vi "reenvioSMS (SubVI).vi"(10 "Datos":T1={"Imei"="359772033694416", "Evento"="359772033694416", "Lat"="359772033694416", "Lon"="359772033694416", "F_H_eve"=timestamp(0 s since 1904-01-01), "F_H_rec"=timestamp(0 s since 1904-01-01)}) -> ()   [LabVIEW 2012]
uses:
  <vilib>/addons/database/Auxilliary.llb/DB Tools Cursor Type.ctl
  <vilib>/addons/database/Connection.llb/DB Tools Open Connec (Path).vi
  <vilib>/addons/database/Connection.llb/Conn Execute.vi
  <vilib>/addons/database/Recordset.llb/Rec Get Recordset Properties (R).vi
  <vilib>/addons/database/Recordset.llb/Rec Fetch String Data (R).vi
  <vilib>/addons/database/Recordset.llb/Rec Destroy - Connection.vi
  <vilib>/addons/database/NI_Database_API.lvlib
panel:
  out "SMS":string
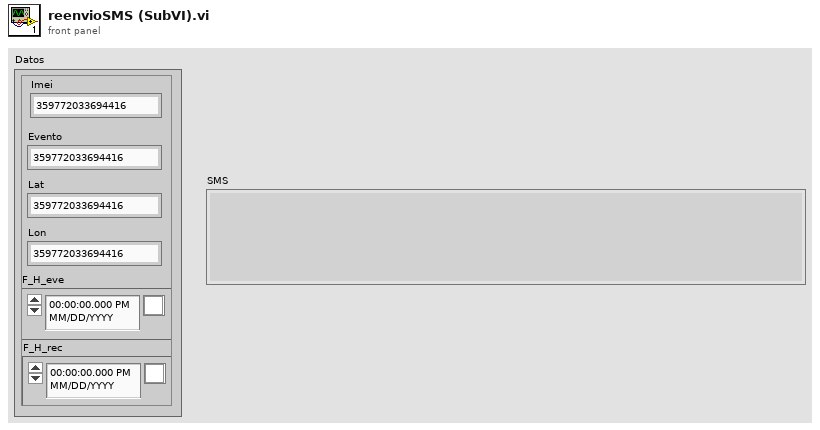
[diagram p1: front panel]
types:
  T1 = cluster{"Imei":string, "Evento":string, "Lat":string, "Lon":string, "F_H_eve":timestamp, "F_H_rec":timestamp}
  T2 = typedef "NI_Database_API.lvlib/DB Tools Cursor Type.ctl" = enum16{"forward-only", "keyset", "dynamic", "static"}
  T3 = enum16{"POC", "Imei", "Evento", "Lat", "Lon", "F_H_eve", "F_H_rec", "AVL_N", "AVL_pass", "Propietario", "Razon_Social", "Direccion", "Propietario_N", "Ciudad", "Marca", "Ruta", "N_Ruta", "Auditor", "Auditor_N"}
  T4 = typedef "NI_Database_API.lvlib/Conn ObjectReference.ctl" = refnum<k1>
  T5 = typedef "NI_Database_API.lvlib/Rec ObjectReference.ctl" = refnum<k1>
  T6 = enum16{"POC", "Imei", "Evento", "Lat", "Lon", "F_H_eve", "F_H_rec", "AVL_N", "AVL_pass", "Propietario", "Razon_Social", "Direccion", "Propietario_N", "Ciudad", "Marca", "Ruta", "N_Ruta", "Auditor_ST", "Auditor_P"}
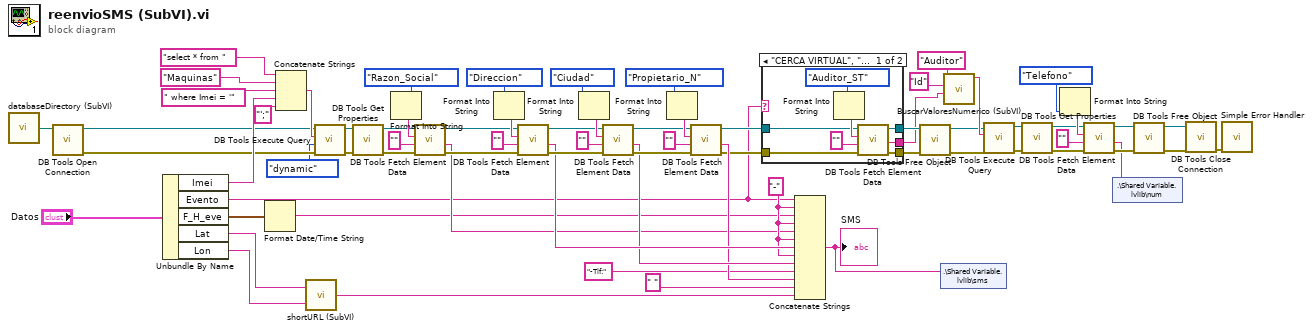
[diagram p0: block diagram]
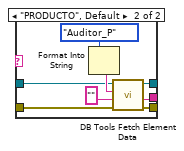
[diagram p2: hidden frame]
diagram:
  w41 = "-" ("type")
  n1 = call "databaseDirectory (SubVI).vi"() -> ("Application Directory"=w38:path)  [unwired: 1 in]
  n2 = call-poly <vilib>:"DB Tools Open Connection.vi"("connection information"=w38) -> ("error out"=w34:errorcluster, "connection reference"=w35:T4)  [unwired: 7 in]
  n3 = Unbundle By Name("Datos") -> ("Imei"=w36:string, "Evento"=w19:string, "F_H_eve"=w29:timestamp, "Lat"=w23:string, "Lon"=w22:string)
  n4 = Format Date/Time String(seconds (now)=w29) -> (date/time string=w28:string)  [unwired: 2 in]
  n5 = Concatenate Strings("select * from " ("SQL query"), "Maquinas" ("table"), " where Imei = '" ("Substring"), w36, "';") -> (w67:string)
  n6 = call "shortURL (SubVI).vi"("LON"=w22, "LAT"=w23) -> ("before substring"=w20:string)
  n7 = call-poly <vilib>:"DB Tools Execute Query.vi"("error in (no error)"=w34, "cursor type"=DB_Tools_Cursor_Type."dynamic", "SQL query"=w67, "connection reference"=w35) -> ("error out"=w68:errorcluster, "recordset reference"=w69:T5)  [unwired: 4 in]
  n8 = call-poly <vilib>:"DB Tools Get Properties.vi"("error in (no error)"=w68, "recordset reference"=w69) -> ("error out"=w26:errorcluster, "recordset reference out"=w27:T5)  [unwired: 3 in, 1 out]
  n9 = Format Into String(T3."Razon_Social") -> (resulting string=w61:string)  [unwired: 3 in, 1 out]
  n10 = call-poly <vilib>:"DB Tools Fetch Element Data.vi"("error in (no error)"=w26, "type"="", "column index"=w61, "recordset reference"=w27) -> ("error out"=w42:errorcluster, "data"=w40:string, "recordset reference out"=w56:T5)  [unwired: 3 in]
  n11 = Format Into String(T3."Direccion") -> (resulting string=w57:string)  [unwired: 3 in, 1 out]
  n12 = call-poly <vilib>:"DB Tools Fetch Element Data.vi"("error in (no error)"=w42, "type"="", "column index"=w57, "recordset reference"=w56) -> ("error out"=w52:errorcluster, "data"=w45:string, "recordset reference out"=w53:T5)  [unwired: 3 in]
  n13 = Format Into String(T3."Ciudad") -> (resulting string=w55:string)  [unwired: 3 in, 1 out]
  n14 = call-poly <vilib>:"DB Tools Fetch Element Data.vi"("error in (no error)"=w52, "type"="", "column index"=w55, "recordset reference"=w53) -> ("error out"=w50:errorcluster, "data"=w44:string, "recordset reference out"=w51:T5)  [unwired: 3 in]
  n15 = Format Into String(T3."Propietario_N") -> (resulting string=w60:string)  [unwired: 3 in, 1 out]
  n16 = call-poly <vilib>:"DB Tools Fetch Element Data.vi"("error in (no error)"=w50, "type"="", "column index"=w60, "recordset reference"=w51) -> ("error out"=w32:errorcluster, "data"=w43:string, "recordset reference out"=w33:T5)  [unwired: 3 in]
  n17 = case shown="\"CERCA VIRTUAL\", \"POC ABIERTO\", \"SERVICIO\"" w19 {
    tunnel: w33 -> [w72 w83]
    tunnel: w32 -> [w71 w82]
    tunnel: [w75 w81] -> w31
    tunnel: [w74 w80] -> w30
    tunnel: [w73 w79] -> w4
    frame "CERCA VIRTUAL", "POC ABIERTO", "SERVICIO" {
      n18 = Format Into String(T6."Auditor_ST") -> (resulting string=w78:string)  [unwired: 3 in, 1 out]
      n19 = call-poly <vilib>:"DB Tools Fetch Element Data.vi"("error in (no error)"=w71, "type"="", "column index"=w78, "recordset reference"=w72) -> ("error out"=w74:errorcluster, "data"=w73:string, "recordset reference out"=w75:T5)  [unwired: 3 in]
    }
    frame "PRODUCTO", Default {
      n20 = Format Into String(T6."Auditor_P") -> (resulting string=w84:string)  [unwired: 3 in, 1 out]
      n21 = call-poly <vilib>:"DB Tools Fetch Element Data.vi"("error in (no error)"=w82, "type"="", "column index"=w84, "recordset reference"=w83) -> ("error out"=w80:errorcluster, "data"=w79:string, "recordset reference out"=w81:T5)  [unwired: 3 in]
    }
  }
  n22 = Concatenate Strings(w19, w41, w28, w41, w40, w41, w45, w41, w44, "-Tlf:" ("type"), w43, " " ("string"), w20) -> (w24:string)
  "SMS" <- w24
  n23 = call-poly <vilib>:"DB Tools Free Object.vi"("error in (no error)"=w30, "recordset reference"=w31) -> ("error out"=w5:errorcluster, "connection reference"=w6:T4)  [unwired: 8 in]
  n24 = shared-variable ".\\Shared Variable.lvlib\\sms"(w24) -> ()  [unwired: 1 in, 1 out]
  n25 = call "BuscarValoresNumerico (SubVI).vi"("="=w4, "Columna"="Id" ("Substring"), "Tabla"="Auditor" ("table")) -> ("String"=w16:string)  [unwired: 8 in]
  n26 = call-poly <vilib>:"DB Tools Execute Query.vi"("error in (no error)"=w5, "SQL query"=w16, "connection reference"=w6) -> ("error out"=w17:errorcluster, "recordset reference"=w18:T5)  [unwired: 5 in]
  n27 = call-poly <vilib>:"DB Tools Get Properties.vi"("error in (no error)"=w17, "recordset reference"=w18) -> ("error out"=w7:errorcluster, "recordset reference out"=w8:T5)  [unwired: 3 in, 1 out]
  n28 = Format Into String(enum16{"Id", "Nombre", "Apellido", "Telefono"}."Telefono") -> (resulting string=w12:string)  [unwired: 3 in, 1 out]
  n29 = call-poly <vilib>:"DB Tools Fetch Element Data.vi"("error in (no error)"=w7, "type"="", "column index"=w12, "recordset reference"=w8) -> ("error out"=w9:errorcluster, "data"=w3:string, "recordset reference out"=w10:T5)  [unwired: 3 in]
  n30 = shared-variable ".\\Shared Variable.lvlib\\num"(w3) -> ()  [unwired: 1 in, 1 out]
  n31 = call-poly <vilib>:"DB Tools Free Object.vi"("error in (no error)"=w9, "recordset reference"=w10) -> ("error out"=w2:errorcluster, "connection reference"=w1:T4)  [unwired: 8 in]
  n32 = call <vilib>:"DB Tools Close Connection.vi"("error in (no error)"=w2, "connection reference"=w1) -> ("error out"=w70:errorcluster)  [unwired: 5 in]
  n33 = call <vilib>:"Simple Error Handler.vi"("error in (no error)"=w70) -> ()  [unwired: 4 in, 5 out]
